vi "2dArrayTo1dArray.vi"(8 "error in (no error)":errorcluster, 10 "2D Array":dbl[][](array[numeric]), 11 "MatOper in":refnum<class "MatOper.lvclass">) -> (0 "error out":errorcluster, 2 "1D Array":dbl[](array[numeric]), 3 "MatOper out":refnum<class "MatOper.lvclass">)   [LabVIEW 2016, in "OfcFunc.lvlib" / "MatOper.lvclass"]
doc: "Reshape the 2D array to 1D array."
uses:
  MatOper.lvclass
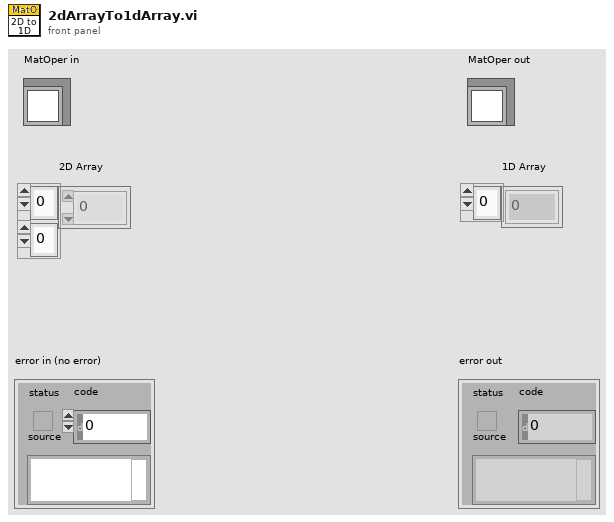
[diagram p1: front panel]
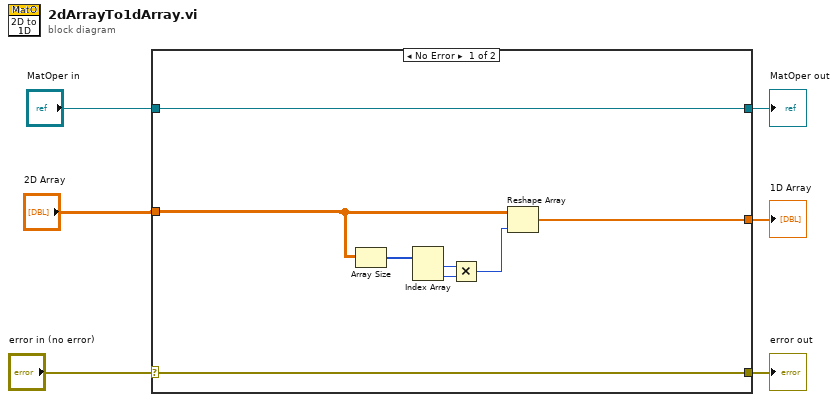
[diagram p0: block diagram]
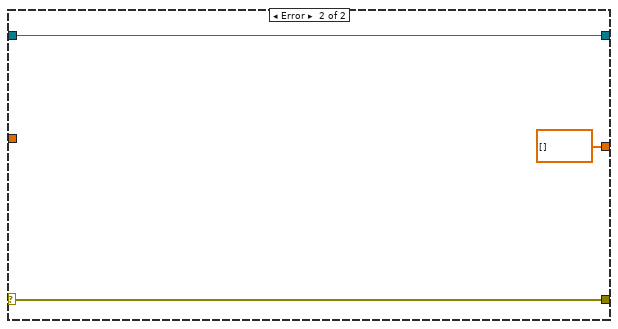
[diagram p2: hidden frame]
diagram:
  n1 = case shown="No Error" "error in (no error)" {
    selector: "error in (no error)" -> [w13 w17]
    tunnel: [w13 w17] -> w5
    tunnel: [w14 w16] -> w3
    tunnel: "MatOper in" -> [w14 w16]
    tunnel: "2D Array" -> [w8 _]
    tunnel: [w7 dbl[] [] ("2D Array")] -> w1
    frame No Error {
      n2 = Array Size(array=w8) -> (size(s)=w12:i32[])
      n3 = Index Array(array=w12) -> (element #1=w10:i32, element #2=w11:i32)  [unwired: 2 in]
      n4 = Multiply(x=w10, y=w11) -> (x*y=w9:i32)
      n5 = Reshape Array(w8, w9) -> (w7:dbl[])
    }
    frame Error {
    }
  }
  "error out" <- w5
  "MatOper out" <- w3
  "1D Array" <- w1
